vi "CTRE_CANifier_GetGeneralInput.vi"(8 "error in":errorcluster, 10 "Input Pin":T1, 11 "CANifierDevRef":T2) -> (0 "error out":errorcluster, 2 "Measured Pin State":bool, 3 "CANifierDevRef":T2)   [LabVIEW 2019]
uses:
  <vilib>/Rock Robotics/WPI/ThirdParty/Phoenix-LabVIEW/CANifier/CTRE_CANifier_DeviceRef.ctl
  <vilib>/Rock Robotics/WPI/ThirdParty/Phoenix-LabVIEW/CANifier/CTRE_CANifier_GeneralPin.ctl
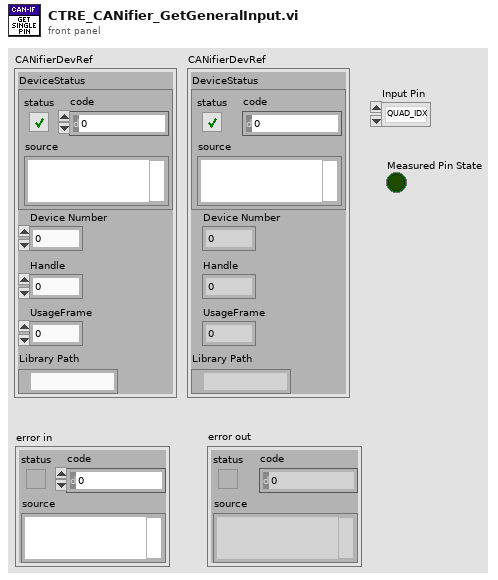
[diagram p1: front panel]
types:
  T1 = typedef "CTRE_CANifier_GeneralPin.ctl" = enum16{"QUAD_IDX", "QUAD_B", "QUAD_A", "LIMR", "LIMF", "SDA", "SCL", "SPI_CS", "SPI_MISO_PWM2", "SPI_MOSI_PWM1", "SPI_CLK_PWM0"}
  T2 = typedef "CTRE_CANifier_DeviceRef.ctl" = cluster{"DeviceStatus":errorcluster, "Device Number":u8, "Handle":u64, "UsageFrame":u32, "Library Path":path}
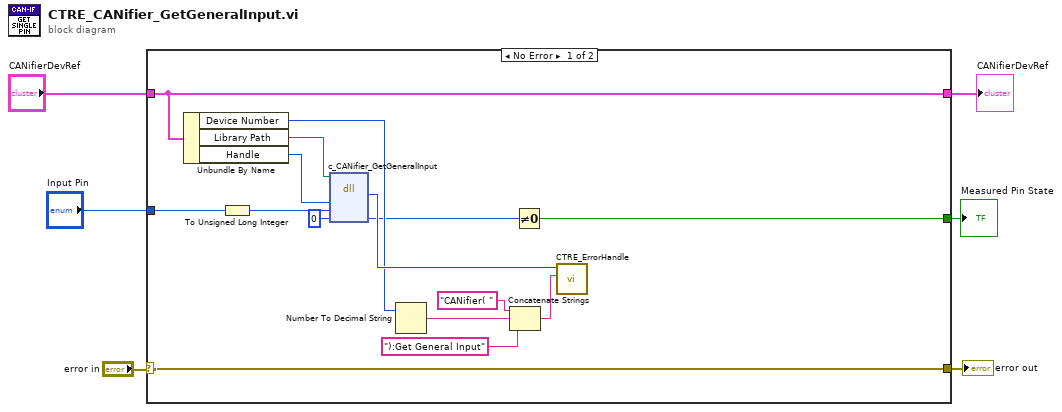
[diagram p0: block diagram]
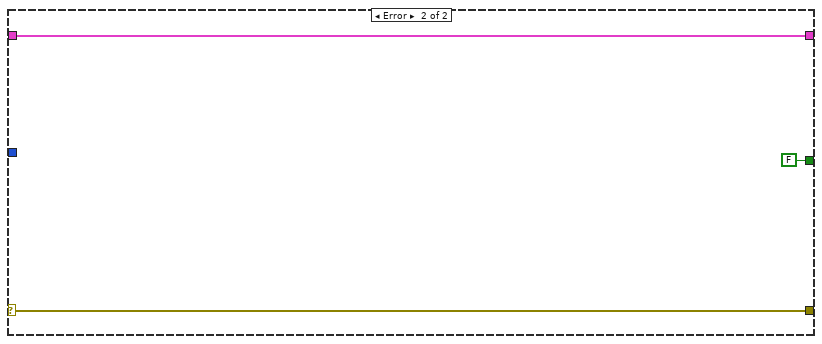
[diagram p2: hidden frame]
diagram:
  n1 = case shown="No Error" "error in" {
    selector: "error in" -> [w21 w24]
    tunnel: [w21 w24] -> w5
    tunnel: "CANifierDevRef" -> [w20 w23]
    tunnel: [w20 w23] -> w3
    tunnel: "Input Pin" -> [w11 _]
    tunnel: [w7 FALSE] -> w1
    frame No Error {
      n2 = Unbundle By Name(w20) -> ("Device Number"=w13:u8, "Library Path"=w19:path, "Handle"=w18:u64)
      n3 = To Unsigned Long Integer(number=w11) -> (unsigned 32bit integer=w10:u32)
      n4 = dll-call lib="?" fn="c_CANifier_GetGeneralInput"(path in=w19, "handle"=w18, "inputPin"=w10, "measuredInput"=u8 0) -> ("CTR_Code"=w17:i8, "measuredInput"=w8:u8)  [unwired: 4 in, 2 out]
      n5 = Number To Decimal String(number=w13) -> (decimal integer string=w16:string)  [unwired: 1 in]
      n6 = Concatenate Strings("CANifier( " ("string"), w16, "):Get General Input" ("string")) -> (w12:string)
      n7 = Not Equal To 0?(x=w8) -> (x != 0?=w7:bool)
      n8 = call <vilib>:"CTRE_ErrorHandle.vi"("origin"=w12, "code"=w17) -> ()  [unwired: 9 in, 1 out]
    }
    frame Error {
    }
  }
  "error out" <- w5
  "CANifierDevRef" <- w3
  "Measured Pin State" <- w1
